vi "UART Read.vi"(8 "Error In":errorcluster, 11 "FPGA Interface":refnum<k20>) -> (0 "Error Out":errorcluster, 1 "UART Console":string, 3 "FPGA Interface Out":refnum<k20>)   [LabVIEW 2015]
uses:
  <vilib>/Utility/error.llb/Error Cluster From Error Code.vi
  <vilib>/rvi/errors/niLvFpgaAdjustHostInterfaceError.vi
  <vilib>/rvi/interface/nirviMethod/nirviMethod.xnode
  <vilib>/FPGAPlugInAG/Dynamic/niLvFpga_ReadFifo_Dynamic.vi
  <vilib>/rvi/errors/niLvFpgaMergeErrorWithErrorCode.vi
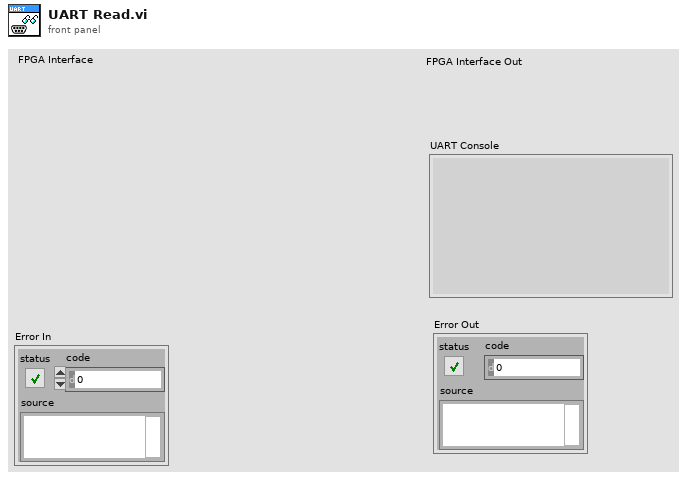
[diagram p1: front panel]
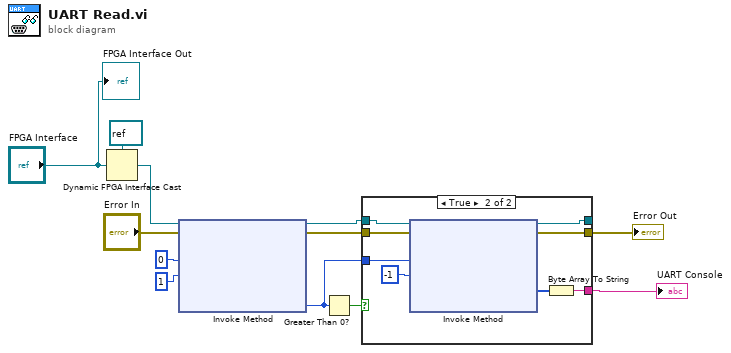
[diagram p0: block diagram]
diagram:
  n1 = Dynamic FPGA Interface Cast(Session In=refnum<k20> refnum ("FPGA Interface"), Type="FPGA Interface") -> (Session Out=w2:refnum<k20>)
  n2 = xnode "Invoke Method"("FPGA VI Reference In"=w2, "error in"="Error In", "Number of Elements"=u32 0, "Timeout (ms)"=1) -> ("FPGA VI Reference Out"=w7:refnum<k20>, "error out"=w8:errorcluster, "Elements Remaining"=w10:u32)  [unwired: 1 out]
  n3 = Greater Than 0?(x=w10) -> (x > 0?=w11:bool)
  n4 = case shown="True" w11 {
    tunnel: w7 -> [w14 w22]
    tunnel: w8 -> [w13 w21]
    tunnel: [w13 w20] -> w12
    tunnel: [w14 w19] -> _
    tunnel: [_ w17] -> w1
    tunnel: w10 -> [_ w16]
    frame False {
    }
    frame True {
      n5 = xnode "Invoke Method"("FPGA VI Reference In"=w22, "error in"=w21, "Number of Elements"=w16, "Timeout (ms)"=-1) -> ("FPGA VI Reference Out"=w19:refnum<k20>, "error out"=w20:errorcluster, "Data"=w18:u16[])  [unwired: 1 out]
      n6 = Byte Array To String(unsigned byte array=w18) -> (string=w17:string)
    }
  }
  "Error Out" <- w12
  "UART Console" <- w1
  "FPGA Interface Out" <- "FPGA Interface"
